vi "Calibrate Position 2 Ticks (uSMC).vi"(1 "array index":i32, 2 "value":dbl) -> (0 "value ticks":i32)   [LabVIEW 2010, in "SignalWriterMH110203USBStepperMotor.lvclass"]
uses:
  SignalWriterMH110203USBStepperMotor.lvclass
  class_data.vi
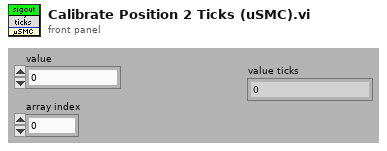
[diagram p1: front panel]
types:
  T1 = typedef "SignalWriterMH110203USBStepperMotor.lvclass/GoTo Control (uSMC).ctl" = cluster{"Step motor ID":string, "SMname":string, "Backlash":u16, "wait for input sygnal to start":bool, "use slow start/stop":bool, "units name":string, "Maximum speed":dbl, "speed":dbl, "step":u8, "point 1 ticks":i32, "point 2 ticks":i32, "point 1 units":dbl, "point 2 units":dbl, "Limit Switch standoff":dbl, "Zero Value":dbl, "Destination Position":dbl, "force backlash":bool, "power off when stop":bool, "POff delay":dbl, "positioner name":string, "R, Ohm":dbl, "I, mA":dbl, "Positioner's Type":u16, "Reset Direction":bool, "Manufacturer":string, "Model":string, "Scheme":string, "FirmwareVer":string}
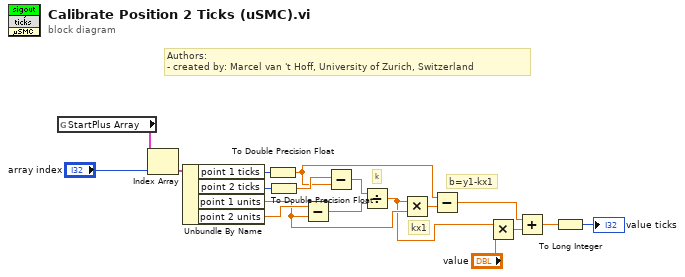
[diagram p0: block diagram]
diagram:
  # "Authors: \n- created by: Marcel van 't Hoff, University of Zurich, Switzerland"
  # "b=y1-kx1"
  # "kx1"
  # "k"
  n1 = global read "class_data.vi" "StartPlus Array"() -> (w18:T1[])
  n2 = Index Array(array=w18, index="array index") -> (element=w16:T1)
  n3 = Unbundle By Name(w16) -> ("point 1 ticks"=w9:i32, "point 2 ticks"=w14:i32, "point 1 units"=w11:dbl, "point 2 units"=w15:dbl)
  n4 = To Double Precision Float(number=w9) -> (double precision float=w2:dbl)
  n5 = To Double Precision Float(number=w14) -> (double precision float=w3:dbl)
  n6 = Subtract(x=w15, y=w11) -> (x-y=w12:dbl)
  n7 = Subtract(x=w3, y=w2) -> (x-y=w13:dbl)
  n8 = Divide(x=w13, y=w12) -> (x/y=w7:dbl)
  n9 = Multiply(x=w7, y=w11) -> (x*y=w10:dbl)
  n10 = Subtract(x=w2, y=w10) -> (x-y=w4:dbl)
  n11 = Multiply(x=w7, y="value") -> (x*y=w5:dbl)
  n12 = Add(x=w4, y=w5) -> (x+y=w1:dbl)
  n13 = To Long Integer(number=w1) -> (32bit integer=→"value ticks":i32)
